vi "Check Distance.vi"(10 "distance":dbl=414.0 format="%#_13g", 11 "Result Arr":T1(array[cluster])) -> (3 "Array":T1(array[cluster]))   [LabVIEW 2019]
panel:
  out "Array 2":dbl[](array[numeric])
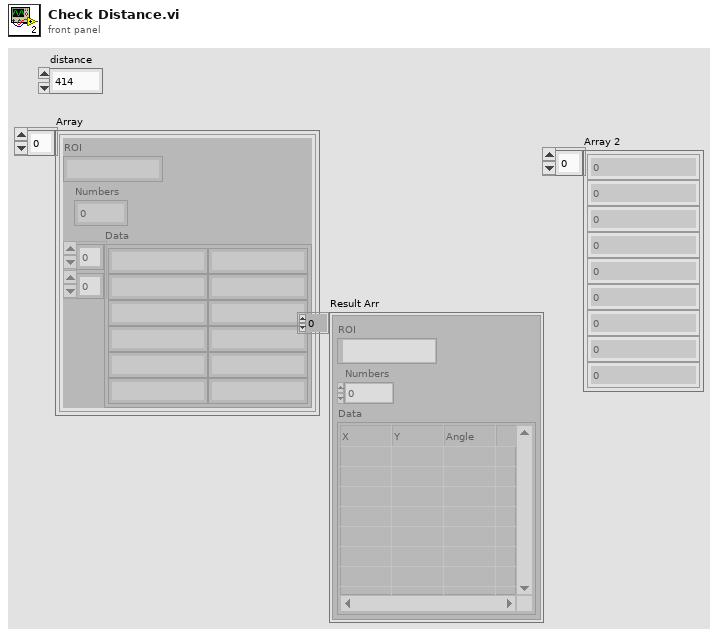
[diagram p1: front panel]
types:
  T1 = cluster{"ROI":string, "Numbers":i32, "Data":string[][]}[]
  T2 = cluster{"ROI":string, "Numbers":i32, "Data":string[][]}
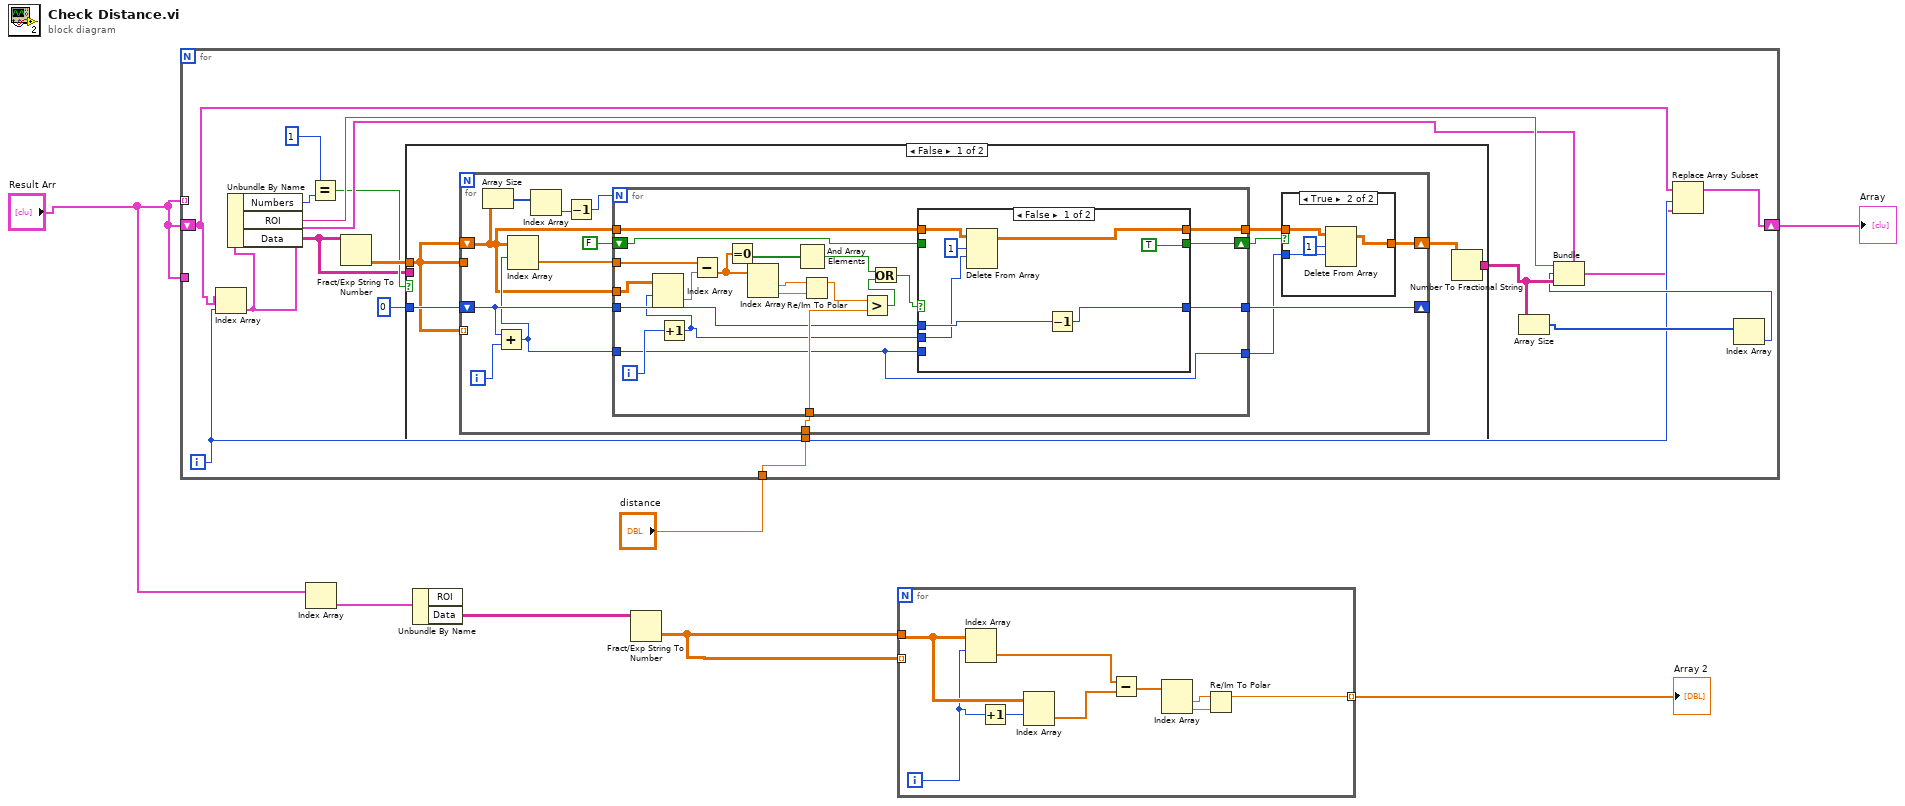
[diagram p0: block diagram]
diagram:
  n1 = for {
    tunnel: "Result Arr" -> [_]
    tunnel: "distance" -> [w23]
    shift-right: [w13] -> w2
    shift-left: "Result Arr" -> [w16]
    tunnel: "Result Arr" -> [_] mode=indexing
    i -> [w15]
    n2 = Index Array(array=w16, index=w15) -> (element=w17:T2)
    n3 = Unbundle By Name(w17) -> ("Numbers"=w11:i32, "ROI"=w18:string, "Data"=w8:string[][])
    n4 = Equal?(x=1, y=w11) -> (x = y?=w9:bool)
    n5 = Fract/Exp String To Number(string=w8) -> (number=w12:dbl[][])  [unwired: 3 in, 1 out]
    n6 = case shown="False" w9 {
      tunnel: w23 -> [w28 _]
      tunnel: 0 -> [w27 _]
      tunnel: [w25 w80] -> w21
      tunnel: w12 -> [w24 _]
      tunnel: w8 -> [_ w80]
      frame False {
        n7 = for {
          tunnel: w24 -> [_]
          tunnel: w28 -> [w42]
          shift-right: [w31] -> w26
          shift-left: w24 -> [w37]
          shift-right: [w39] -> _
          shift-left: w27 -> [w40]
          tunnel: w24 -> [_] mode=indexing
          i -> [w41]
          n8 = Array Size(array=w37) -> (size(s)=w36:i32[])
          n9 = Add(x=w40, y=w41) -> (x+y=w38:i32)
          n10 = Index Array(array=w37, index (row)=w38) -> (element=w43:dbl[])  [unwired: 1 in]
          n11 = Index Array(array=w36) -> (element=w35:i32)  [unwired: 1 in]
          n12 = Decrement(x=w35) -> (x-1=w34:i32)
          n13 = for {
            N: w34 -> [_]
            tunnel: w43 -> [w69]
            tunnel: w37 -> [w60]
            tunnel: w37 -> [w63]
            tunnel: w42 -> [w65]
            tunnel: [w64] -> w32
            tunnel: w40 -> [w62]
            tunnel: [w61] -> w39
            tunnel: w38 -> [w49]
            shift-right: [w50] -> w30
            shift-left: FALSE -> [w51]
            tunnel: [w49] -> w29
            i -> [w59]
            n14 = Increment(x=w59) -> (x+1=w57:i32)
            n15 = Index Array(array=w60, index (row)=w57) -> (element=w58:dbl[])  [unwired: 1 in]
            n16 = Subtract(x=w69, y=w58) -> (x-y=w56:dbl[])
            n17 = Equal To 0?(x=w56) -> (x = 0?=w55:bool[])
            n18 = Index Array(array=w56) -> (element #1=w68:dbl, element #2=w67:dbl)  [unwired: 2 in]
            n19 = And Array Elements(Boolean array=w55) -> (logical AND=w53:bool)
            n20 = Re/Im To Polar(2:w67, 3:w68) -> (1:w66:dbl)  [unwired: 1 out]
            n21 = Greater?(x=w66, y=w65) -> (0:w54:bool)
            n22 = Or(x=w53, y=w54) -> (x .or. y?=w52:bool)
            n23 = case shown="False" w52 {
              tunnel: [w71 w79] -> w64
              tunnel: w63 -> [w74 w79]
              tunnel: w62 -> [w76 w78]
              tunnel: [w75 w78] -> w61
              tunnel: w57 -> [w73 _]
              tunnel: w49 -> [_ _]
              tunnel: w51 -> [_ w77]
              tunnel: [TRUE w77] -> w50
              frame False {
                n24 = Delete From Array(array=w74, length=1, index (row)=w73) -> (array with subset deleted=w71:dbl[][])  [unwired: 1 in, 1 out]
                n25 = Decrement(x=w76) -> (x-1=w75:i32)
              }
              frame True {
              }
            }
          }
          n26 = case shown="True" w30 {
            tunnel: w32 -> [w44 w48]
            tunnel: [w44 w47] -> w31
            tunnel: w29 -> [_ w46]
            frame False {
            }
            frame True {
              n27 = Delete From Array(array=w48, length=1, index (row)=w46) -> (array with subset deleted=w47:dbl[][])  [unwired: 1 in, 1 out]
            }
          }
        }
        n28 = Number To Fractional String(number=w26) -> (F-format string=w25:string[][])  [unwired: 3 in]
      }
      frame True {
      }
    }
    n29 = Array Size(array=w21) -> (size(s)=w20:i32[])
    n30 = Index Array(array=w20) -> (element=w19:i32)  [unwired: 1 in]
    n31 = Bundle(cluster=w17, "ROI"=w18, "Numbers"=w19, "Data"=w21) -> (w14:T2)
    n32 = Replace Array Subset(array=w16, new element=w14, index=w15) -> (w13:T1)
  }
  "Array" <- w2
  n33 = Index Array(array="Result Arr") -> (element=w6:T2)  [unwired: 1 in]
  n34 = Unbundle By Name(w6) -> ("Data"=w5:string[][])  [unwired: 1 out]
  n35 = Fract/Exp String To Number(string=w5) -> (number=w3:dbl[][])  [unwired: 3 in, 1 out]
  n36 = for {
    tunnel: w3 -> [w89]
    tunnel: [w81] -> w4 mode=indexing
    tunnel: w3 -> [_] mode=indexing
    i -> [w88]
    n37 = Index Array(array=w89, index (row)=w88) -> (element=w83:dbl[])  [unwired: 1 in]
    n38 = Increment(x=w88) -> (x+1=w87:i32)
    n39 = Index Array(array=w89, index (row)=w87) -> (element=w82:dbl[])  [unwired: 1 in]
    n40 = Subtract(x=w83, y=w82) -> (x-y=w84:dbl[])
    n41 = Index Array(array=w84) -> (element #1=w86:dbl, element #2=w85:dbl)  [unwired: 2 in]
    n42 = Re/Im To Polar(2:w85, 3:w86) -> (1:w81:dbl)  [unwired: 1 out]
  }
  "Array 2" <- w4
